vi "excel.vi"(0 "1d array":dbl[](array[numeric]), 3 "Sheet name":string="10k1k") -> ()   [LabVIEW 2014]
panel:
  in  "empty":dbl[](array[numeric])
  out "2d array":dbl[][](array[numeric])
  in  "error in (no error)":errorcluster
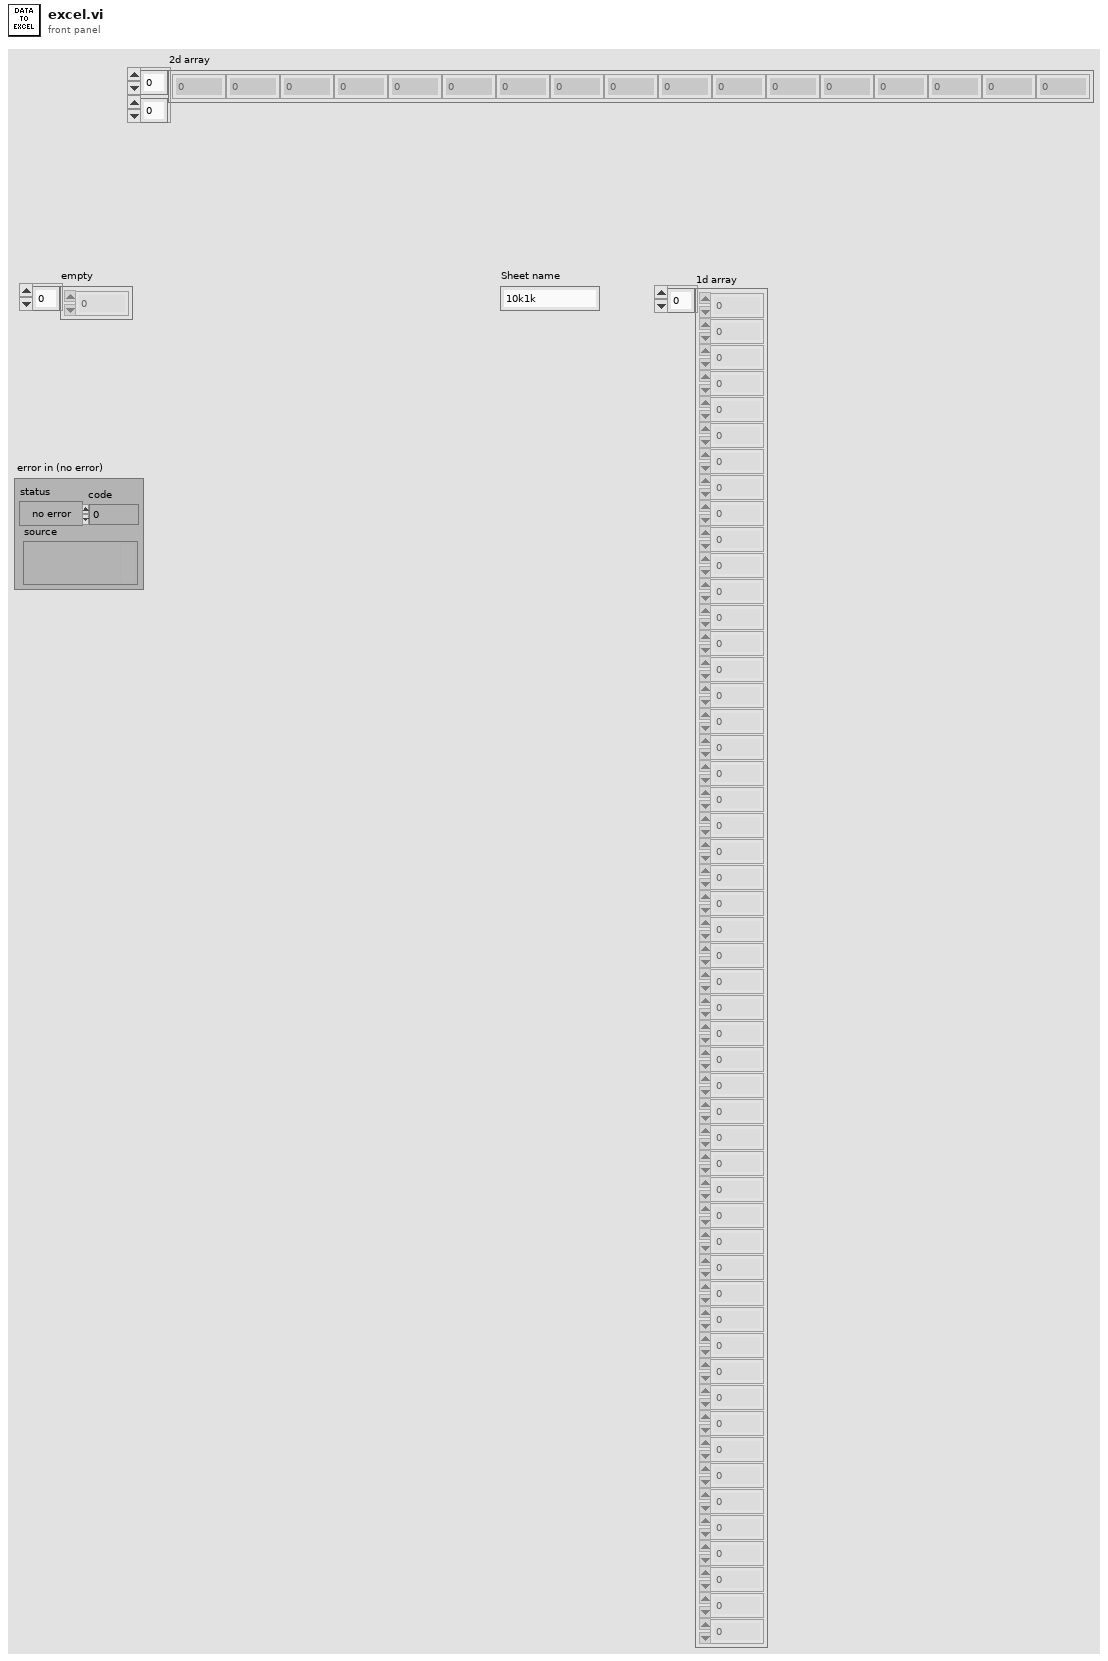
[diagram p1: front panel]
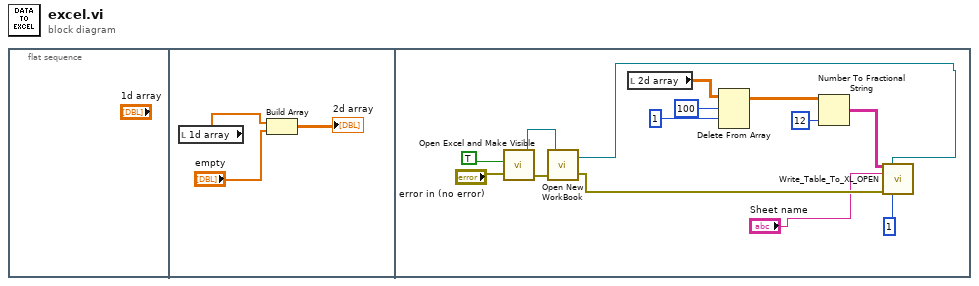
[diagram p0: block diagram]
diagram:
  n1 = flat-sequence {
    frame #0 {
    }
    frame #1 {
      n2 = local read "1d array"() -> (w3:dbl[])
      n3 = Build Array(w3, "empty") -> (→"2d array":dbl[][])
    }
    frame #2 {
      n4 = call "Open Excel and Make Visible.vi"("error in (no error)"="error in (no error)", "Visible Boolean"=TRUE) -> ("error out"=w14:errorcluster, "Excel._Application"=w15:refnum<k7>)
      n5 = call "Open New  WorkBook.vi"("error in (no error)"=w14, "Excel._Application"=w15) -> ("error out"=w10:errorcluster, "Excel._Workbook"=w11:refnum<k7>)  [unwired: 1 out]
      n6 = local read "2d array"() -> (w7:dbl[][])
      n7 = Delete From Array(array=w7, length=100, index (row)=1) -> (array with subset deleted=w4:dbl[][])  [unwired: 1 in, 1 out]
      n8 = Number To Fractional String(number=w4, precision (6)=i16 12) -> (F-format string=w16:string[][])  [unwired: 2 in]
      n9 = call "Write_Table_To_XL_OPEN.vi"("Table"=w16, "Excel._Workbook"=w11, "SheetName"="Sheet name", "error in (no error)"=w10, "Page index"=1) -> ()  [unwired: 10 in, 1 out]
    }
  }
